vi "MonitorICL.vi"(8 "error in":errorcluster, 9 "Show Frontpanel?":bool, 10 "Event Registration Refnum":refnum<event-registration>, 11 "DeviceManager in":refnum<class "DeviceManager.lvclass">) -> (0 "error out":errorcluster, 3 "DeviceManager out":refnum<class "DeviceManager.lvclass">)   [LabVIEW 2023, in "DeviceManager.lvclass"]
uses:
  DeviceManager.lvclass
  DeviceManager.lvclass/DeviceManager.ctl
panel:
  out "ICL output":string caption="StdErr"
  out "StdOut":string
  # "Locals"
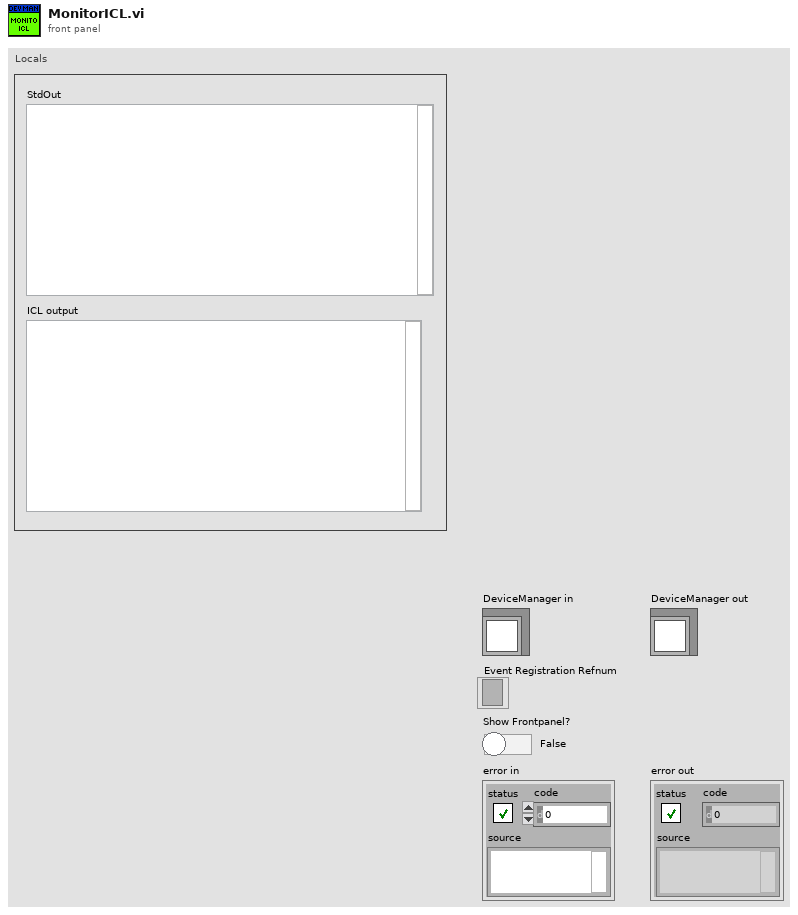
[diagram p1: front panel]
types:
  T1 = enum32{"Invalid", "Standard", "Closed", "Hidden", "Minimized", "Maximized"}
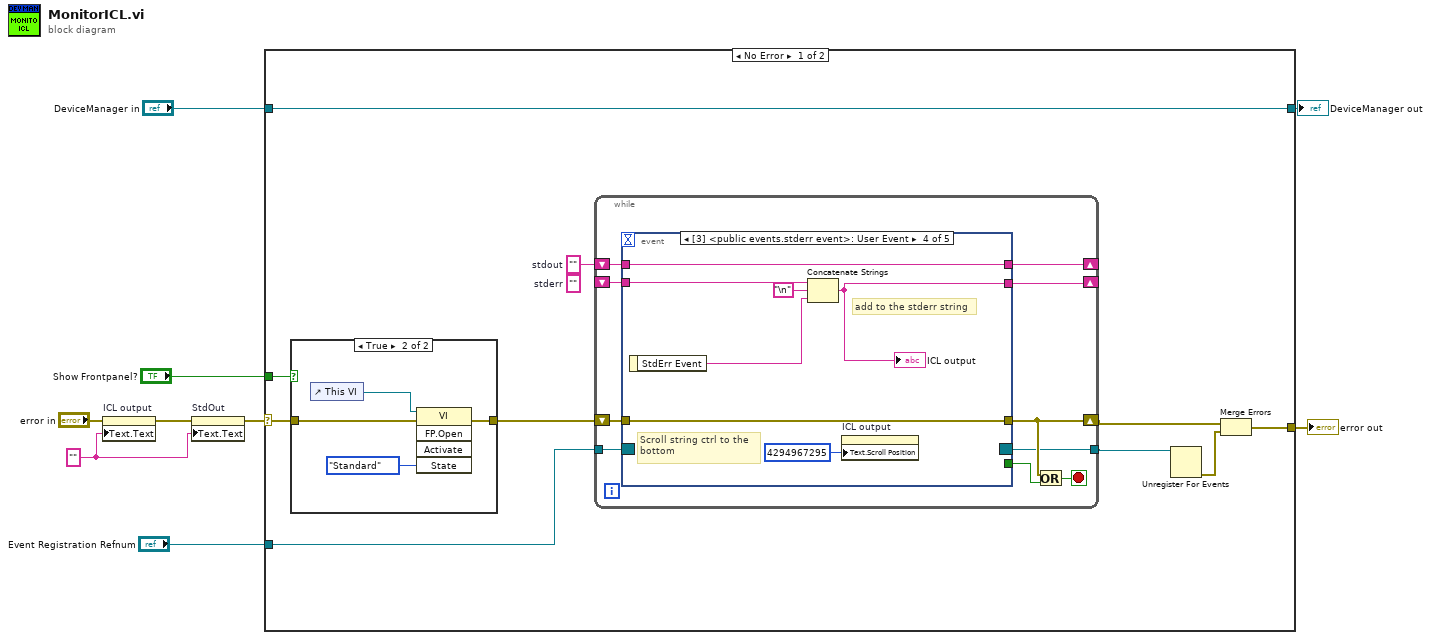
[diagram p0: block diagram]
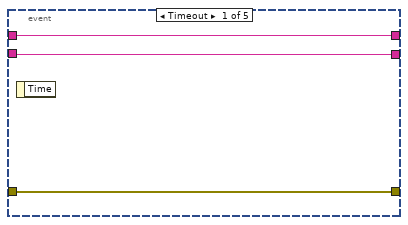
[diagram p3: hidden frame]
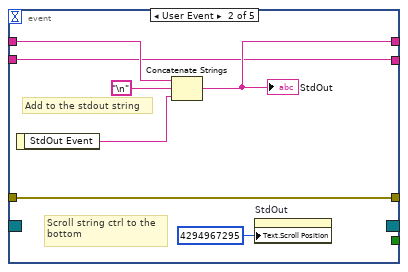
[diagram p4: hidden frame]
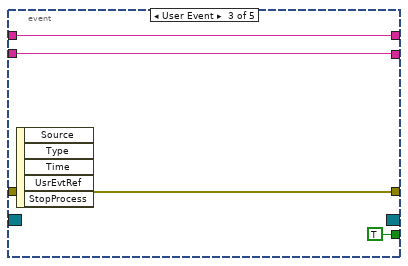
[diagram p5: hidden frame]
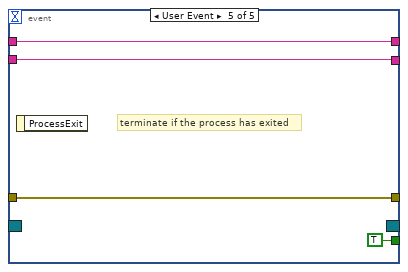
[diagram p6: hidden frame]
diagram:
  w1 = "" ("Text.Text")
  n1 = property on="ICL output" class="Str"(error in="error in", "Text.Text"=w1) -> (error out=w2:errorcluster)  [unwired: 1 in, 1 out]
  n2 = property on="StdOut" class="Str"(error in=w2, "Text.Text"=w1) -> (error out=w4:errorcluster)  [unwired: 1 in, 1 out]
  n3 = case shown="No Error" w4 {
    selector: w4 -> [w12 w61]
    tunnel: [w18 w61] -> w9
    tunnel: [w13 w60] -> w7
    tunnel: "DeviceManager in" -> [w13 w60]
    tunnel: "Event Registration Refnum" -> [w15 _]
    tunnel: "Show Frontpanel?" -> [w10 _]
    frame No Error {
      (unwired) ""  # stderr
      w16 = ""  # stdout
      n4 = case shown="True" w10 {
        tunnel: w12 -> [w20 w24]
        tunnel: [w20 w23] -> w11
        frame False {
        }
        frame True {
          n5 = control-ref of="This VI"() -> (w21:refnum<vi>)
          n6 = invoke class="VI" method="FP.Open"(reference=w21, error in=w24, "State"=T1."Standard") -> (error out=w23:errorcluster)  [unwired: 2 in, 4 out]
        }
      }
      n7 = while {
        shift-right: [w33] -> w17
        shift-left: w11 -> [w34]
        tunnel: w15 -> [w32]
        tunnel: [w31] -> w14
        shift-right: [w29] -> _
        shift-left: w16 -> [w30]
        shift-right: [w27] -> _
        shift-left: _ -> [w28]
        stop <- w26 stop-if-true
        n8 = event shown="[3] <public events.stderr event>: User Event" {
          selector: w32 -> [_ _ _ _ _]
          dyn-events: [_ _ _ _ _] -> w31
          timeout: _ -> [_ _ _ _ _]
          tunnel: w34 -> [w37 w44 w48 w55 w59]
          tunnel: [w37 w44 w48 w55 w59] -> w33
          tunnel: w30 -> [w36 w41 w47 w51 w57]
          tunnel: [w36 w42 w47 w51 w57] -> w29
          tunnel: [_ _ TRUE ("ProcessExit") _ TRUE ("ProcessExit")] -> w25
          tunnel: w28 -> [w35 w39 w46 w52 w58]
          tunnel: [w35 w39 w46 w50 w58] -> w27
          event Timeout {
            n9 = event-data() -> ()  [unwired: 1 in, 1 out]
          }
          event User Event {
            # "Scroll string ctrl to the \nbottom"
            # "Add to the stdout string"
            n10 = event-data() -> ("StdOut Event"=w40:string)  [unwired: 1 in]
            n11 = Concatenate Strings(w41, "\n", w40) -> (w42:string)
            "StdOut" <- w42
            n12 = property on="StdOut" class="Str"("Text.Scroll Position"=u32 4294967295) -> ()  [unwired: 2 in, 2 out]
          }
          event User Event {
            n13 = event-data() -> ()  [unwired: 1 in, 5 out]
          }
          event User Event {
            # "Scroll string ctrl to the \nbottom"
            # "add to the stderr string"
            n14 = event-data() -> ("StdErr Event"=w53:string)  [unwired: 1 in]
            n15 = Concatenate Strings(w52, "\n", w53) -> (w50:string)
            "ICL output" <- w50
            n16 = property on="ICL output" class="Str"("Text.Scroll Position"=u32 4294967295) -> ()  [unwired: 2 in, 2 out]
          }
          event User Event {
            # "terminate if the process has exited"
            n17 = event-data() -> ()  [unwired: 1 in, 1 out]
          }
        }
        n18 = Or(x=w33, y=w25) -> (x .or. y?=w26:bool)
      }
      n19 = Unregister For Events(event registration refnum=w14) -> (error out=w19:errorcluster)  [unwired: 1 in]
      n20 = Merge Errors(w17, w19) -> (w18:errorcluster)
    }
    frame Error {
    }
  }
  "error out" <- w9
  "DeviceManager out" <- w7
